vi "Microphone Filter.vi"() -> ()   [LabVIEW 2015]
doc: "The myRIO Project template acquires acceleration data from the onboard accelerometer and displays the changes of acceleration values in a waveform chart."
uses:
  <vilib>/myRIO/Instrument Drivers/Onboard IO/AI/AI.lvlib
  <vilib>/myRIO/Instrument Drivers/Utilities/Utilities.lvlib
  <vilib>/Analysis/NI_AALBase.lvlib
  <vilib>/Analysis/3filter.llb/Butterworth Filter (DBL).vi
  <vilib>/Analysis/3filter.llb/Filter Passband Type.ctl
panel:
  in  "low cutoff freq: fl 2":dbl=0.12500000000000006 format="%0.4f"
  in  "high cutoff freq: fh 2":dbl=0.45000000000000007 format="%0.2f"
  in  "filter type 3":T1
  in  "filter type 2":T1
  in  "high cutoff freq: fh":dbl=0.45000000000000007 format="%0.2f"
  out "error":i32
  in  "low cutoff freq: fl":dbl=0.12500000000000006 format="%0.4f"
  in  "filter type":T1
  out "Waveform Chart 2":dbl[](graph)
  in  "Stop":bool
  out "Waveform Chart":dbl[](graph)
  # "Overview: The myRIO Project template acquires acceleration data from the onboard accelerometer and displays the changes of acceleration values in a waveform chart.\nInstructions:\n1. Check the myRIO target IP address in the project and make sure the target IP address is correct. \n2. Run this VI."
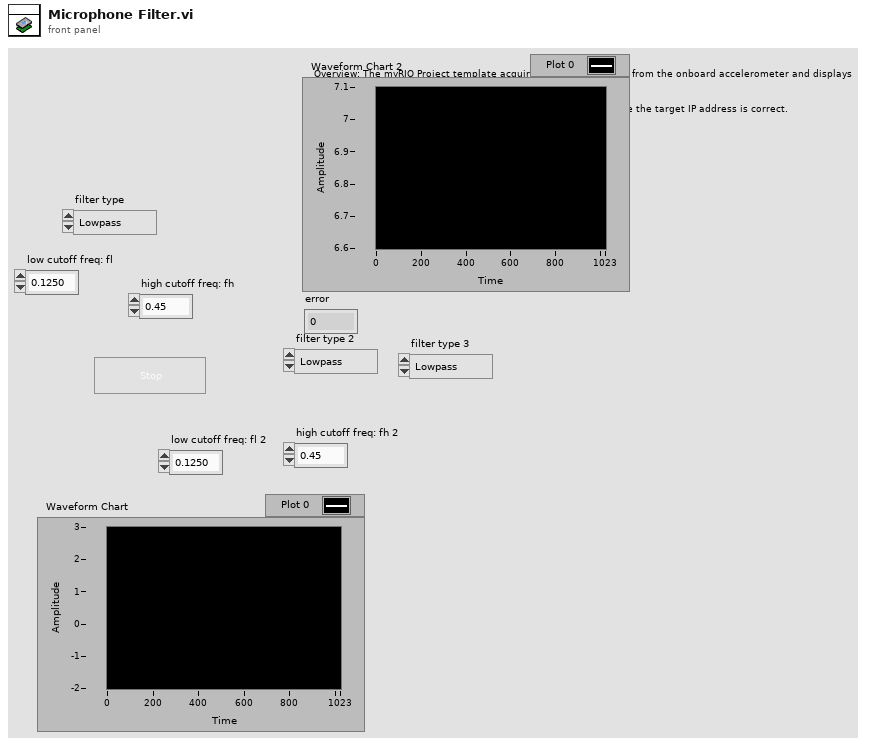
[diagram p1: front panel]
types:
  T1 = typedef "NI_AALBase.lvlib/Filter Passband Type.ctl" = enum32{"Lowpass", "Highpass", "Bandpass", "Bandstop"}
  T2 = typedef "AI.lvlib/AI Reference.ctl" = cluster{"myRIO Reference":T3, "AI Channels List":T7, "AI Scaling Constants List":T9}
  T3 = typedef "myRIO Generic Hardware Reference.ctl" = cluster{"myRIO Model":T4, "myRIO Hardware Reference":T5}
  T4 = typedef "Hardware Version Enum.ctl" = enum16{"Unknown", "myRIO-1900", "myRIO-1950", "roboRIO"}
  T5 = typedef "myRIO v1.0 Reference.ctl" = cluster{"Generic FPGA Reference":T6, "Allow multiple opens":bool}
  T6 = typedef "Generic FPGA Reference.ctl" = refnum<k20>
  T7 = typedef "AI Channels List.ctl" = T8[]
  T8 = typedef "AI Channels Enum.ctl" = enum16{"Not Connected", "AudioIn/Left", "AudioIn/Right", "C/AI0", "C/AI1", "A/AI0", "A/AI1", "A/AI2", "A/AI3", "B/AI0", "B/AI1", "B/AI2", "B/AI3", "AI/AI0", "AI/AI1", "AI/AI2", "AI/AI3"}
  T9 = typedef "Analog Scaling Constants List.ctl" = T10[]
  T10 = typedef "Analog Scaling Constants.ctl" = cluster{"LSB Weight (Volts)":dbl, "Offset (Volts)":dbl, "Signed?":bool}
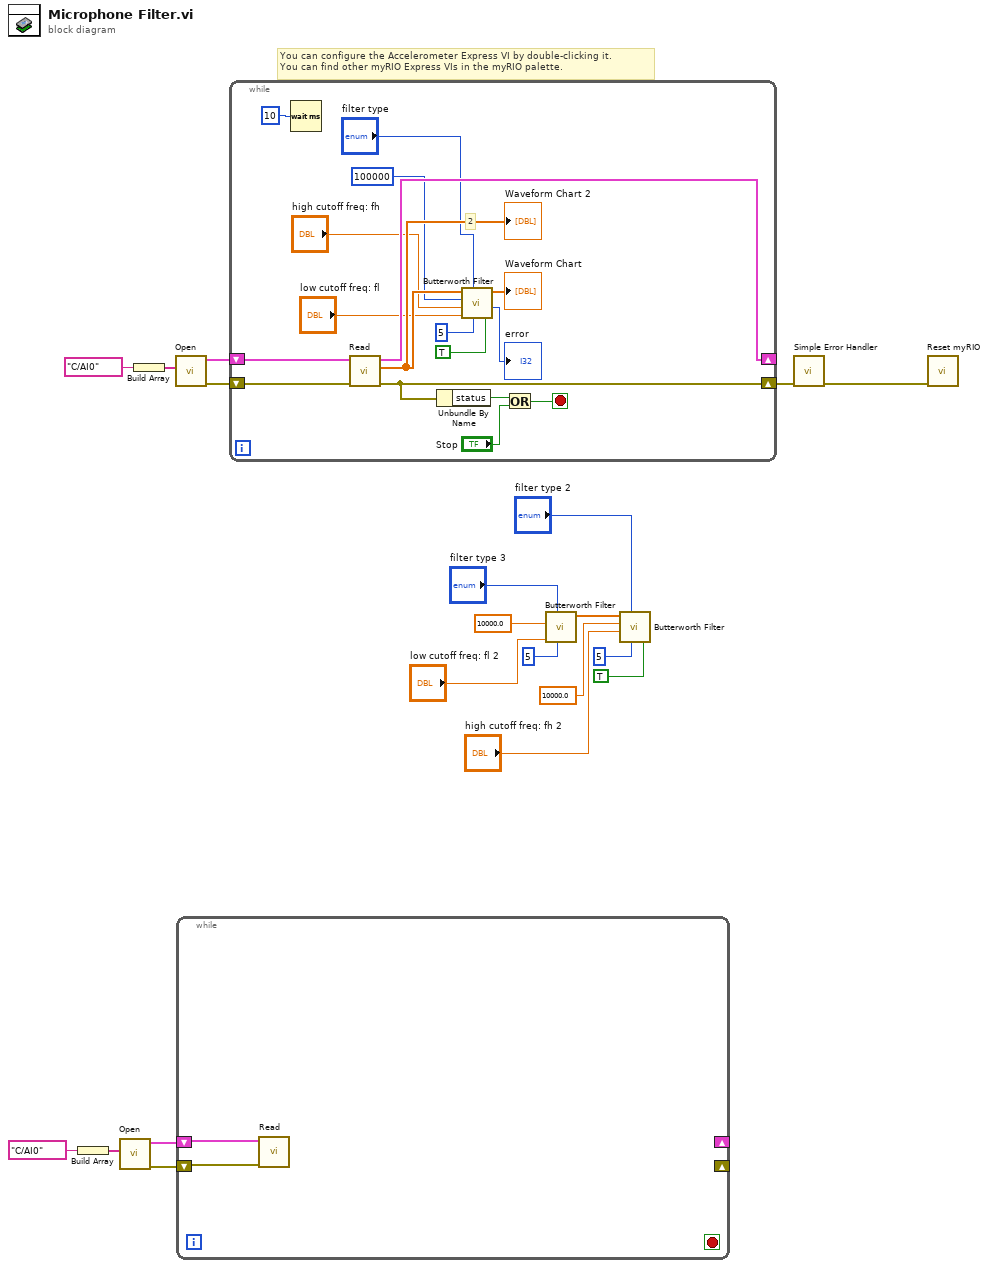
[diagram p0: block diagram]
diagram:
  # "You can configure the Accelerometer Express VI by double-clicking it.\nYou can find other myRIO Express VIs in the myRIO palette."
  n1 = Build Array(tag "C/AI0" ("myRIO AI Channel")) -> (w3:tag[])
  n2 = call <vilib>:"Open.vi"("Channel Names"=w3) -> ("error out"=w1:errorcluster, "AI Ref Out"=w2:T2)  [unwired: 9 in]
  n3 = Build Array(tag "C/AI0" ("myRIO AI Channel")) -> (w19:tag[])
  n4 = call <vilib>:"Open.vi"("Channel Names"=w19) -> ("error out"=w17:errorcluster, "AI Ref Out"=w18:T2)  [unwired: 9 in]
  n5 = while {
    shift-right: _ -> [_]
    shift-left: w2 -> [w22]
    shift-right: _ -> [_]
    shift-left: w1 -> [w21]
    stop <- _ stop-if-true
    n6 = call <vilib>:"Read.vi"("error in (no error)"=w21, "AI Ref In"=w22) -> ()  [unwired: 7 in, 3 out]
  }
  n7 = while {
    shift-right: [w34] -> _
    shift-left: w18 -> [w35]
    shift-right: [w33] -> w15
    shift-left: w17 -> [w36]
    stop <- w39 stop-if-true
    # "2"
    n8 = Wait (ms)(milliseconds to wait=10) -> ()  [unwired: 1 out]
    n9 = call <vilib>:"Read.vi"("error in (no error)"=w36, "AI Ref In"=w35) -> ("error out"=w33:errorcluster, "Values"=w30:dbl[], "AI Ref Out"=w34:T2)  [unwired: 7 in]
    "Waveform Chart 2" <- w30
    n10 = Unbundle By Name(w33) -> ("status"=w38:bool)
    n11 = call-poly <vilib>:"Butterworth Filter.vi"("init/cont (init:F)"=TRUE, "order"=5, "filter type"="filter type", "low cutoff freq: fl"="low cutoff freq: fl", "high cutoff freq: fh"="high cutoff freq: fh", "sampling freq: fs"=100000, "X"=w30) -> ("error"=→"error":i32, "Filtered X"=→"Waveform Chart":dbl[])  [unwired: 1 in]
    n12 = Or(x=w38, y="Stop") -> (x .or. y?=w39:bool)
  }
  n13 = call-poly <vilib>:"Butterworth Filter.vi"("order"=5, "filter type"="filter type 3", "low cutoff freq: fl"="low cutoff freq: fl 2", "sampling freq: fs"=10000.0) -> ("Filtered X"=w6:dbl[])  [unwired: 4 in, 1 out]
  n14 = call-poly <vilib>:"Butterworth Filter.vi"("init/cont (init:F)"=TRUE, "order"=5, "filter type"="filter type 2", "high cutoff freq: fh"="high cutoff freq: fh 2", "sampling freq: fs"=10000.0, "X"=w6) -> ()  [unwired: 2 in, 2 out]
  n15 = call <vilib>:"Simple Error Handler.vi"("error in (no error)"=w15) -> ("error out"=w16:errorcluster)  [unwired: 4 in, 4 out]
  n16 = call <vilib>:"Reset myRIO.vi"("error in (no error)"=w16) -> ()  [unwired: 10 in, 1 out]
